vi "Read TrayStatus.vi"(8 "error in (no error)":errorcluster, 10 "F1/T2":bool, 11 "AI in":refnum<class "AI.lvclass">) -> (0 "error out":errorcluster, 1 "Arr_TrayST":bool[][](array[boolean]), 2 "Arr_Tray":cluster{"X":sgl, "Y":sgl}[][](array[cluster]), 3 "AI out":refnum<class "AI.lvclass">)   [LabVIEW 2019, in "AI.lvclass"]
uses:
  AI.lvclass
  Function/TraySet Folder/global/Tray_ArrAndData.vi
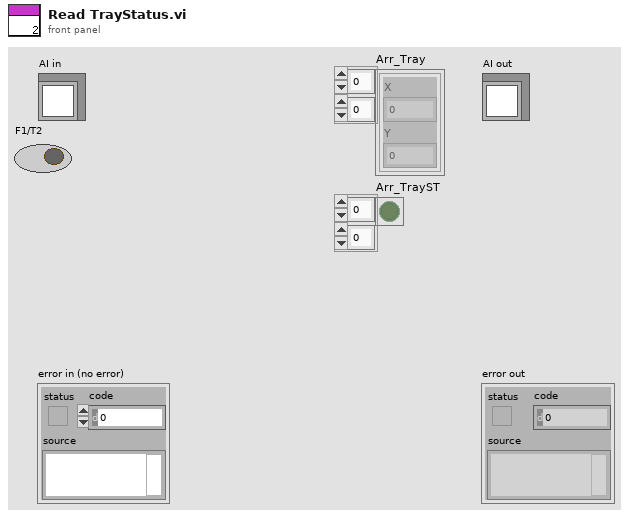
[diagram p1: front panel]
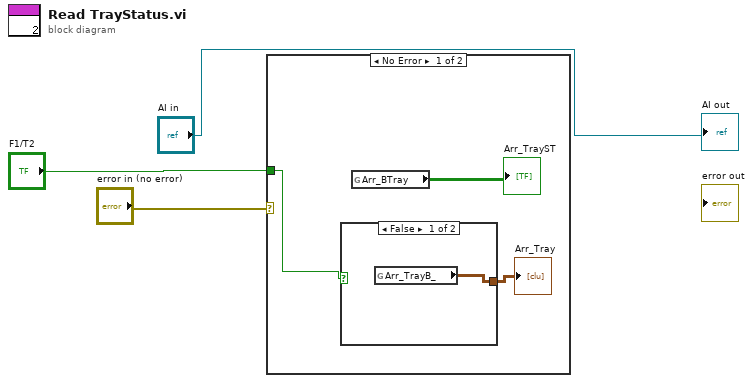
[diagram p0: block diagram]
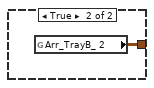
[diagram p2: hidden frame]
diagram:
  n1 = case shown="No Error" "error in (no error)" {
    tunnel: "F1/T2" -> [w6 _]
    frame No Error {
      n2 = case shown="False" w6 {
        tunnel: [w7 w8] -> w4
        frame False {
          n3 = global read "Tray_ArrAndData.vi" "Arr_TrayB_"() -> (w7:cluster{"X":sgl, "Y":sgl}[][])
        }
        frame True {
          n4 = global read "Tray_ArrAndData.vi" "Arr_TrayB_ 2"() -> (w8:cluster{"X":sgl, "Y":sgl}[][])
        }
      }
      "Arr_Tray" <- w4
      n5 = global read "Tray_ArrAndData.vi" "Arr_BTray"() -> (→"Arr_TrayST":bool[][])
    }
    frame Error {
    }
  }
  "AI out" <- "AI in"
